vi "冰箱设置.vi"() -> ()   [LabVIEW 2016, in "采配水.lvlib"]
uses:
  <vilib>/Utility/config.llb/NI_LVConfig.lvlib
panel:
  in  "关闭时间":u16(ring)=2 items=["00H", "01H", "02H", "03H", "04H", "05H", "06H", "07H", "08H", "09H", "10H", "11H", "12H", "13H", "14H", "15H", "16H", "17H", "18H", "19H", "20H", "21H", "22H", "23H", "关闭"]
  in  "功能开关":enum16{"关闭", "开启"}(ring)
  in  "开启时间":u16(ring)=2 items=["00H", "01H", "02H", "03H", "04H", "05H", "06H", "07H", "08H", "09H", "10H", "11H", "12H", "13H", "14H", "15H", "16H", "17H", "18H", "19H", "20H", "21H", "22H", "23H", "关闭"]
  in  "布尔":bool
  # "参数设置"
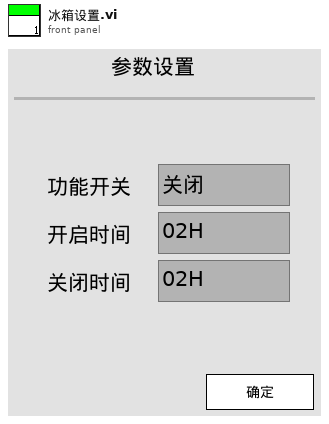
[diagram p1: front panel]
types:
  T1 = cluster{"功能开关":enum16{"关闭", "开启"}, "开启时间":u16, "关闭时间":u16}
  T2 = typedef "NI_LVConfig.lvlib/Config Data RefNum.ctl" = refnum<k1>
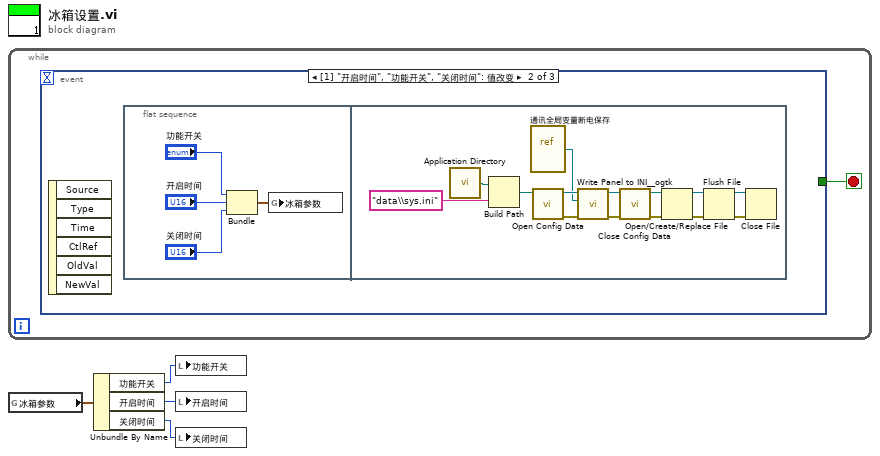
[diagram p0: block diagram]
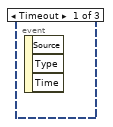
[diagram p2: hidden frame]
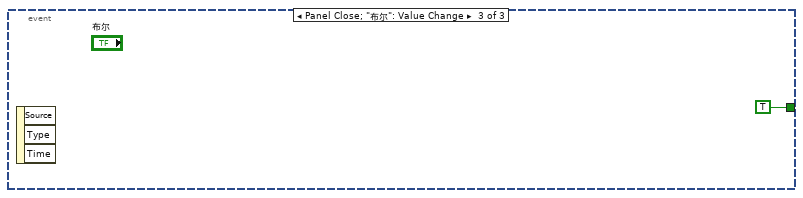
[diagram p3: hidden frame]
diagram:
  n1 = while {
    stop <- w5 stop-if-true
    n2 = event shown="[1] \"开启时间\", \"功能开关\", \"关闭时间\": 值改变" {
      selector: _ -> [_ _ _]
      dyn-events: _ -> [_ _ _]
      timeout: _ -> [_ _ _]
      tunnel: [_ _ TRUE] -> w5
      event Timeout {
        n3 = event-data() -> ()  [unwired: 1 in, 3 out]
      }
      event "开启时间", "功能开关", "关闭时间": Value Change {
        n4 = event-data() -> ()  [unwired: 1 in, 6 out]
        n5 = flat-sequence {
          frame #0 {
            n6 = Bundle("功能开关"="功能开关", "开启时间"="开启时间", "关闭时间"="关闭时间") -> (w9:T1)  [unwired: 1 in]
            n7 = global write "通讯全局变量断电保存.vi" "冰箱参数"(w9) -> ()
          }
          frame #1 {
            n8 = call <vilib>:"Application Directory.vi"() -> ("Application Directory"=w23:path)
            n9 = Build Path(base path=w23, name or relative path="data\\sys.ini" ("名称或相对路径")) -> (appended path=w21:path)
            n10 = vi-ref "通讯全局变量断电保存.vi"() -> (w19:refnum<vi>)
            n11 = call <vilib>:"Open Config Data.vi"("configuration file path"=w21) -> ("error out"=w17:errorcluster, "refnum"=w20:T2)  [unwired: 8 in, 1 out]
            n12 = call <userlib>:"Write Panel to INI__ogtk.vi"("error in (no error)"=w17, "VI ref"=w19, "refnum"=w20) -> ("error out"=w16:errorcluster, "refnum out"=w18:T2)  [unwired: 7 in]
            n13 = call <vilib>:"Close Config Data.vi"("error in (no error)"=w16, "refnum"=w18) -> ("error out"=w11:errorcluster, "file path"=w10:path)  [unwired: 8 in]
            n14 = Open/Create/Replace File(file path (use dialog)=w10, error in=w11) -> (refnum out=w14:refnum<file>, error out=w15:errorcluster)  [unwired: 4 in, 1 out]
            n15 = Flush File(refnum=w14, error in=w15) -> (refnum out=w13:refnum<file>, error out=w12:errorcluster)
            n16 = Close File(refnum=w13, error in=w12) -> ()  [unwired: 2 out]
          }
        }
      }
      event Panel Close; "布尔": Value Change {
        n17 = event-data() -> ()  [unwired: 1 in, 3 out]
      }
    }
  }
  n18 = global read "通讯全局变量断电保存.vi" "冰箱参数"() -> (w4:T1)
  n19 = Unbundle By Name(w4) -> ("功能开关"=w3:enum16{"关闭", "开启"}, "开启时间"=w1:u16, "关闭时间"=w2:u16)
  n20 = local write "功能开关"(w3) -> ()
  n21 = local write "开启时间"(w1) -> ()
  n22 = local write "关闭时间"(w2) -> ()
